vi "initialConf.vi"(10 "VISA":refnum<visa-resource-name>, 11 "ElectrometerConfiguration.lvclass":refnum<class "ElectrometerConfiguration.lvclass">) -> (3 "ElectrometerConfiguration":refnum<class "ElectrometerConfiguration.lvclass">)   [LabVIEW 2016]
uses:
  ElectrometerConfiguration.lvclass
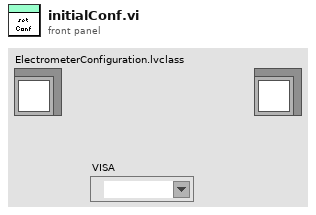
[diagram p1: front panel]
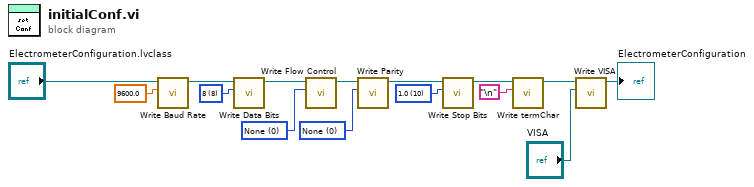
[diagram p0: block diagram]
diagram:
  w4 = u16 10 items=["1.0"=10, "1.5"=15, "2.0"=20] ("Stop Bits")
  w5 = u16 0 items=["None", "Odd", "Even", "Mark", "Space"] ("Parity")
  w6 = u16 0 items=["None", "XON/XOFF", "RTS/CTS", "XON/XOFF & RTS/CTS", "DTR/DSR", "XON/XOFF & DTR/DSR"] ("Flow Control")
  w7 = u16 8 items=["7"=7, "8"=8] ("Data Bits")
  n1 = call-dynamic "Write Baud Rate.vi"("Baud Rate"=9600.0, "ElectrometerConfiguration in"="ElectrometerConfiguration.lvclass") -> ("ElectrometerConfiguration out"=w15:refnum<class "ElectrometerConfiguration.lvclass">)  [unwired: 8 in, 1 out]
  n2 = call-dynamic "Write Data Bits.vi"("Data Bits"=w7, "ElectrometerConfiguration in"=w15) -> ("ElectrometerConfiguration out"=w14:refnum<class "ElectrometerConfiguration.lvclass">)  [unwired: 8 in, 1 out]
  n3 = call-dynamic "Write Flow Control.vi"("Flow Control"=w6, "ElectrometerConfiguration in"=w14) -> ("ElectrometerConfiguration out"=w13:refnum<class "ElectrometerConfiguration.lvclass">)  [unwired: 8 in, 1 out]
  n4 = call-dynamic "Write Parity.vi"("Parity"=w5, "ElectrometerConfiguration in"=w13) -> ("ElectrometerConfiguration out"=w12:refnum<class "ElectrometerConfiguration.lvclass">)  [unwired: 8 in, 1 out]
  n5 = call-dynamic "Write Stop Bits.vi"("Stop Bits"=w4, "ElectrometerConfiguration in"=w12) -> ("ElectrometerConfiguration out"=w11:refnum<class "ElectrometerConfiguration.lvclass">)  [unwired: 8 in, 1 out]
  n6 = call-dynamic "Write termChar.vi"("termChar"="\n", "ElectrometerConfiguration in"=w11) -> ("ElectrometerConfiguration out"=w10:refnum<class "ElectrometerConfiguration.lvclass">)  [unwired: 8 in, 1 out]
  n7 = call-dynamic "Write VISA.vi"("VISA"="VISA", "ElectrometerConfiguration in"=w10) -> ("ElectrometerConfiguration out"=→"ElectrometerConfiguration":refnum<class "ElectrometerConfiguration.lvclass">)  [unwired: 8 in, 1 out]
